vi "Day 5.vi"() -> ()   [LabVIEW 2023]
uses:
  <vilib>/Utility/error.llb/Trim Whitespace One-Sided.vi
panel:
  in  "CrateMover 9001":bool
  out "cargo":string[][](array[string])
  out "i":string
  out "giant cargo crane":string[](array[string])
  out "Top stack answer":string
  out "Moves":string[](array[string])
  in  "input":string="[B]                     [N]     [H]\n[V]         [P] [T]     [V]     [P]\n[W]     [C] [T] [S]     [H]     [N]\n[T]     [J] [Z] [M] [N] [F]     [L]\n[Q]     [W] [N] [J] [T] [Q] [R] [B]\n[N] [B] [Q] [R] [V] [F] [D] [F] [M]\n[H] [W] [S] [J] [P] [W] [L] [P] [S]\n[D] [D] [T] [F] [G] [B] [B] [H] [Z]\n 1   2   3   4   5   6   7   8   9 \n\nmove 2 from 8 to 1\nmove 4 from 9 to 8\nmove 2 from 1 to 6\nmove 7 from 4 to 2\nmove 10 from 2 to 7\nmove 2 from 1 to 6\nmove 1 from 9 to 4\nmove 1 from 4 to 1\nmove 8 from 6 to 4\nmove 7 from 1 to 8\nmove 6 from 8 to 1\nmove 1 from 4 to 1\nmove 8 from 7 to 3\nmove 2 from 5 to 2\nmove 5 from 3 to 2\nmove 5 from 2 to 1\nmove 1 from 6 to 5\nmove 2 from 2 to 6\nmove 5 from 8 to 7\nmove 12 from 7 to 4\nmove 3 from 5 to 4\nmove 2 from 6 to 4\nmove 9 from 1 to 7\nmove 4 from 3 to 7\nmove 4 from 3 to 4\nmove 3 from 1 to 7\nmove 1 from 9 to 1\nmove 1 from 1 to 4\nmove 2 from 5 to 2\nmove 1 from 3 to 7\nmove 15 from 7 to 2\nmove 4 from 7 to 9\nmove 6 from 9 to 2\nmove 2 from 8 to 3\nmove 3 from 2 to 8\nmove 1 from 7 to 6\nmove 8 from 2 to 5\nmove 2 from 8 to 4\nmove 2 from 3 to 8\nmove 9 from 5 to 9\nmove 7 from 4 to 2\nmove 1 from 8 to 6\nmove 6 from 9 to 2\nmove 3 from 9 to 7\nmove 2 from 8 to 4\nmove 7 from 2 to 6\nmove 7 from 4 to 1\nmove 3 from 1 to 8\nmove 2 from 1 to 8\nmove 4 from 8 to 2\nmove 2 from 1 to 5\nmove 19 from 2 to 7\nmove 8 from 4 to 7\nmove 18 from 7 to 1\nmove 11 from 7 to 4\nmove 15 from 1 to 7\nmove 9 from 4 to 3\nmove 2 from 3 to 1\nmove 9 from 4 to 5\nmove 1 from 8 to 1\nmove 8 from 6 to 5\nmove 3 from 2 to 5\nmove 1 from 6 to 7\nmove 4 from 4 to 3\nmove 8 from 5 to 1\nmove 13 from 1 to 6\nmove 12 from 7 to 1\nmove 12 from 6 to 3\nmove 1 from 7 to 6\nmove 1 from 7 to 5\nmove 1 from 1 to 9\nmove 1 from 3 to 1\nmove 3 from 1 to 9\nmove 12 from 3 to 8\nmove 1 from 9 to 3\nmove 1 from 6 to 8\nmove 5 from 5 to 1\nmove 1 from 6 to 2\nmove 10 from 8 to 9\nmove 13 from 9 to 2\nmove 10 from 3 to 4\nmove 1 from 8 to 9\nmove 2 from 8 to 7\nmove 1 from 3 to 1\nmove 1 from 5 to 6\nmove 13 from 2 to 5\nmove 1 from 9 to 2\nmove 7 from 1 to 4\nmove 2 from 2 to 5\nmove 2 from 7 to 8\nmove 1 from 6 to 8\nmove 10 from 5 to 8\nmove 3 from 7 to 2\nmove 4 from 1 to 4\nmove 12 from 4 to 2\nmove 10 from 5 to 3\nmove 6 from 2 to 1\nmove 2 from 4 to 8\nmove 3 from 4 to 8\nmove 6 from 1 to 7\nmove 1 from 7 to 5\nmove 12 from 8 to 2\nmove 3 from 4 to 9\nmove 1 from 4 to 3\nmove 2 from 9 to 6\nmove 2 from 6 to 8\nmove 1 from 1 to 3\nmove 8 from 2 to 6\nmove 4 from 1 to 8\nmove 12 from 2 to 3\nmove 4 from 6 to 8\nmove 10 from 8 to 3\nmove 14 from 3 to 8\nmove 5 from 5 to 8\nmove 1 from 7 to 8\nmove 5 from 3 to 5\nmove 4 from 7 to 2\nmove 2 from 6 to 1\nmove 4 from 3 to 7\nmove 4 from 5 to 1\nmove 21 from 8 to 6\nmove 7 from 3 to 2\nmove 1 from 5 to 1\nmove 4 from 8 to 9\nmove 16 from 6 to 1\nmove 1 from 8 to 4\nmove 5 from 9 to 2\nmove 7 from 1 to 7\nmove 10 from 1 to 3\nmove 1 from 4 to 2\nmove 6 from 6 to 5\nmove 6 from 1 to 4\nmove 4 from 7 to 9\nmove 1 from 6 to 5\nmove 5 from 7 to 6\nmove 3 from 6 to 8\nmove 1 from 7 to 6\nmove 6 from 4 to 8\nmove 4 from 8 to 3\nmove 4 from 8 to 4\nmove 17 from 2 to 1\nmove 8 from 3 to 4\nmove 5 from 4 to 3\nmove 10 from 1 to 5\nmove 11 from 3 to 5\nmove 1 from 7 to 9\nmove 3 from 6 to 4\nmove 9 from 4 to 9\nmove 7 from 1 to 3\nmove 1 from 4 to 8\nmove 7 from 5 to 4\nmove 18 from 5 to 1\nmove 13 from 1 to 6\nmove 1 from 1 to 5\nmove 1 from 1 to 6\nmove 2 from 3 to 1\nmove 1 from 3 to 1\nmove 5 from 1 to 6\nmove 4 from 5 to 8\nmove 2 from 4 to 9\nmove 1 from 1 to 9\nmove 6 from 3 to 8\nmove 1 from 4 to 5\nmove 10 from 8 to 7\nmove 16 from 6 to 7\nmove 1 from 5 to 4\nmove 1 from 7 to 2\nmove 2 from 2 to 6\nmove 2 from 8 to 5\nmove 5 from 4 to 9\nmove 2 from 5 to 9\nmove 7 from 9 to 8\nmove 2 from 6 to 9\nmove 4 from 8 to 9\nmove 7 from 9 to 7\nmove 13 from 9 to 5\nmove 10 from 5 to 1\nmove 3 from 8 to 4\nmove 5 from 1 to 3\nmove 3 from 5 to 6\nmove 3 from 9 to 7\nmove 1 from 1 to 7\nmove 2 from 1 to 3\nmove 1 from 6 to 1\nmove 4 from 3 to 8\nmove 1 from 8 to 9\nmove 1 from 8 to 7\nmove 1 from 8 to 4\nmove 1 from 9 to 7\nmove 1 from 8 to 5\nmove 2 from 4 to 3\nmove 4 from 6 to 3\nmove 1 from 5 to 1\nmove 1 from 6 to 4\nmove 2 from 4 to 5\nmove 1 from 4 to 6\nmove 1 from 6 to 4\nmove 30 from 7 to 3\nmove 1 from 5 to 1\nmove 6 from 7 to 3\nmove 2 from 1 to 7\nmove 2 from 1 to 2\nmove 2 from 2 to 1\nmove 1 from 4 to 9\nmove 3 from 1 to 2\nmove 1 from 9 to 5\nmove 2 from 7 to 1\nmove 1 from 7 to 3\nmove 1 from 1 to 9\nmove 1 from 5 to 8\nmove 1 from 1 to 2\nmove 1 from 7 to 3\nmove 1 from 9 to 4\nmove 18 from 3 to 4\nmove 1 from 5 to 9\nmove 1 from 9 to 6\nmove 1 from 2 to 7\nmove 1 from 8 to 7\nmove 1 from 6 to 3\nmove 1 from 7 to 2\nmove 14 from 4 to 6\nmove 1 from 7 to 6\nmove 15 from 6 to 4\nmove 20 from 3 to 1\nmove 5 from 4 to 9\nmove 5 from 4 to 2\nmove 15 from 1 to 7\nmove 11 from 7 to 9\nmove 2 from 7 to 6\nmove 1 from 6 to 4\nmove 1 from 6 to 3\nmove 2 from 7 to 8\nmove 10 from 4 to 3\nmove 15 from 9 to 3\nmove 1 from 9 to 7\nmove 29 from 3 to 6\nmove 3 from 1 to 6\nmove 1 from 8 to 4\nmove 2 from 4 to 3\nmove 1 from 8 to 9\nmove 4 from 6 to 1\nmove 20 from 6 to 2\nmove 5 from 1 to 9\nmove 3 from 6 to 2\nmove 4 from 6 to 3\nmove 4 from 3 to 1\nmove 4 from 1 to 4\nmove 3 from 4 to 8\nmove 6 from 3 to 4\nmove 6 from 2 to 6\nmove 1 from 7 to 1\nmove 3 from 6 to 8\nmove 6 from 9 to 3\nmove 1 from 1 to 4\nmove 1 from 1 to 7\nmove 3 from 4 to 5\nmove 2 from 6 to 4\nmove 2 from 5 to 6\nmove 4 from 8 to 7\nmove 1 from 5 to 6\nmove 1 from 8 to 4\nmove 1 from 8 to 4\nmove 2 from 4 to 9\nmove 4 from 7 to 8\nmove 4 from 4 to 3\nmove 1 from 7 to 9\nmove 4 from 8 to 6\nmove 1 from 3 to 4\nmove 1 from 3 to 5\nmove 2 from 4 to 7\nmove 4 from 6 to 3\nmove 2 from 9 to 1\nmove 2 from 7 to 4\nmove 1 from 5 to 1\nmove 1 from 3 to 4\nmove 1 from 9 to 3\nmove 4 from 4 to 5\nmove 2 from 5 to 3\nmove 1 from 5 to 7\nmove 1 from 5 to 8\nmove 2 from 6 to 4\nmove 3 from 1 to 3\nmove 21 from 3 to 5\nmove 3 from 6 to 1\nmove 1 from 7 to 1\nmove 4 from 2 to 6\nmove 1 from 8 to 2\nmove 10 from 2 to 4\nmove 4 from 1 to 2\nmove 1 from 6 to 5\nmove 2 from 6 to 9\nmove 7 from 4 to 9\nmove 1 from 6 to 5\nmove 3 from 9 to 4\nmove 6 from 2 to 8\nmove 3 from 9 to 1\nmove 8 from 4 to 3\nmove 1 from 9 to 4\nmove 21 from 5 to 7\nmove 1 from 1 to 3\nmove 2 from 9 to 6\nmove 14 from 7 to 1\nmove 2 from 4 to 1\nmove 2 from 8 to 7\nmove 1 from 8 to 2\nmove 11 from 2 to 9\nmove 8 from 9 to 6\nmove 4 from 7 to 1\nmove 1 from 7 to 4\nmove 2 from 3 to 5\nmove 1 from 1 to 6\nmove 1 from 8 to 2\nmove 3 from 7 to 5\nmove 6 from 1 to 7\nmove 1 from 8 to 7\nmove 1 from 4 to 5\nmove 4 from 6 to 5\nmove 6 from 7 to 6\nmove 3 from 9 to 1\nmove 1 from 7 to 3\nmove 11 from 5 to 1\nmove 1 from 5 to 2\nmove 9 from 6 to 4\nmove 1 from 7 to 3\nmove 2 from 6 to 1\nmove 1 from 2 to 1\nmove 1 from 2 to 6\nmove 14 from 1 to 5\nmove 1 from 8 to 4\nmove 10 from 1 to 5\nmove 3 from 5 to 1\nmove 8 from 3 to 8\nmove 16 from 5 to 7\nmove 2 from 1 to 9\nmove 3 from 8 to 1\nmove 1 from 2 to 4\nmove 6 from 7 to 4\nmove 3 from 5 to 8\nmove 2 from 3 to 6\nmove 7 from 1 to 7\nmove 14 from 4 to 3\nmove 9 from 7 to 8\nmove 2 from 4 to 1\nmove 9 from 8 to 4\nmove 7 from 8 to 2\nmove 6 from 1 to 8\nmove 1 from 9 to 7\nmove 1 from 1 to 6\nmove 1 from 9 to 6\nmove 1 from 5 to 9\nmove 1 from 5 to 3\nmove 9 from 4 to 9\nmove 3 from 3 to 6\nmove 8 from 6 to 3\nmove 1 from 2 to 9\nmove 8 from 9 to 8\nmove 6 from 2 to 9\nmove 2 from 6 to 1\nmove 7 from 8 to 6\nmove 2 from 9 to 6\nmove 8 from 7 to 8\nmove 1 from 4 to 5\nmove 9 from 3 to 5\nmove 2 from 1 to 4\nmove 1 from 7 to 4\nmove 2 from 4 to 3\nmove 11 from 8 to 1\nmove 1 from 4 to 7\nmove 1 from 7 to 8\nmove 5 from 1 to 3\nmove 4 from 6 to 4\nmove 2 from 4 to 8\nmove 1 from 4 to 8\nmove 7 from 8 to 9\nmove 1 from 8 to 9\nmove 1 from 8 to 5\nmove 18 from 3 to 2\nmove 17 from 2 to 7\nmove 6 from 5 to 4\nmove 1 from 2 to 5\nmove 4 from 4 to 6\nmove 4 from 6 to 9\nmove 15 from 7 to 9\nmove 2 from 1 to 6\nmove 2 from 7 to 9\nmove 28 from 9 to 2\nmove 1 from 6 to 7\nmove 4 from 6 to 9\nmove 3 from 1 to 7\nmove 2 from 6 to 3\nmove 1 from 4 to 7\nmove 8 from 9 to 5\nmove 13 from 5 to 3\nmove 1 from 5 to 7\nmove 3 from 9 to 4\nmove 8 from 3 to 7\nmove 28 from 2 to 5\nmove 1 from 9 to 8\nmove 4 from 3 to 4\nmove 4 from 7 to 5\nmove 2 from 3 to 9\nmove 21 from 5 to 4\nmove 1 from 5 to 7\nmove 1 from 3 to 5\nmove 3 from 5 to 7\nmove 1 from 1 to 3\nmove 3 from 7 to 3\nmove 5 from 7 to 6\nmove 10 from 4 to 8\nmove 6 from 5 to 4\nmove 1 from 9 to 3\nmove 15 from 4 to 5\nmove 10 from 4 to 7\nmove 3 from 3 to 7\nmove 1 from 3 to 4\nmove 1 from 3 to 4\nmove 7 from 5 to 1\nmove 2 from 4 to 7\nmove 1 from 9 to 2\nmove 2 from 6 to 9\nmove 1 from 5 to 3\nmove 1 from 3 to 8\nmove 10 from 7 to 9\nmove 2 from 8 to 1\nmove 9 from 9 to 2\nmove 1 from 4 to 3\nmove 9 from 8 to 7\nmove 1 from 2 to 8\nmove 5 from 5 to 4\nmove 1 from 3 to 2\nmove 5 from 4 to 3\nmove 3 from 5 to 9\nmove 6 from 7 to 3\nmove 1 from 6 to 5\nmove 5 from 9 to 7\nmove 2 from 5 to 6\nmove 3 from 6 to 7\nmove 4 from 1 to 4\nmove 6 from 2 to 7\nmove 17 from 7 to 5\nmove 1 from 6 to 1\nmove 5 from 3 to 6\nmove 10 from 7 to 2\nmove 1 from 8 to 4\nmove 1 from 9 to 8\nmove 3 from 4 to 1\nmove 1 from 7 to 4\nmove 5 from 5 to 9\nmove 2 from 8 to 7\nmove 3 from 3 to 7\nmove 4 from 2 to 3\nmove 3 from 4 to 6\nmove 7 from 5 to 8\nmove 7 from 2 to 8\nmove 4 from 9 to 8\nmove 12 from 8 to 3\nmove 17 from 3 to 2\nmove 1 from 7 to 9\nmove 1 from 3 to 9\nmove 3 from 9 to 1\nmove 2 from 5 to 1\nmove 1 from 3 to 5\nmove 4 from 5 to 8\nmove 6 from 8 to 1\nmove 17 from 2 to 3\nmove 13 from 3 to 2\nmove 1 from 3 to 9\nmove 1 from 8 to 4\nmove 1 from 4 to 8\nmove 1 from 9 to 1\nmove 2 from 7 to 2\nmove 8 from 6 to 2\nmove 2 from 7 to 5\nmove 9 from 1 to 3\nmove 13 from 2 to 9\nmove 6 from 1 to 4\nmove 6 from 4 to 5\nmove 3 from 8 to 1\nmove 2 from 1 to 8\nmove 8 from 5 to 7\nmove 2 from 3 to 1\nmove 9 from 3 to 1\nmove 3 from 8 to 2\nmove 1 from 1 to 9\nmove 1 from 3 to 9\nmove 6 from 7 to 3\nmove 4 from 2 to 7\nmove 14 from 1 to 6\nmove 2 from 3 to 9\nmove 3 from 3 to 7\nmove 6 from 2 to 1\nmove 2 from 1 to 2\nmove 9 from 6 to 3\nmove 11 from 9 to 5\nmove 9 from 7 to 6\nmove 6 from 6 to 2\nmove 1 from 1 to 8\nmove 5 from 9 to 4\nmove 1 from 8 to 5\nmove 9 from 2 to 7\nmove 10 from 5 to 8\n"
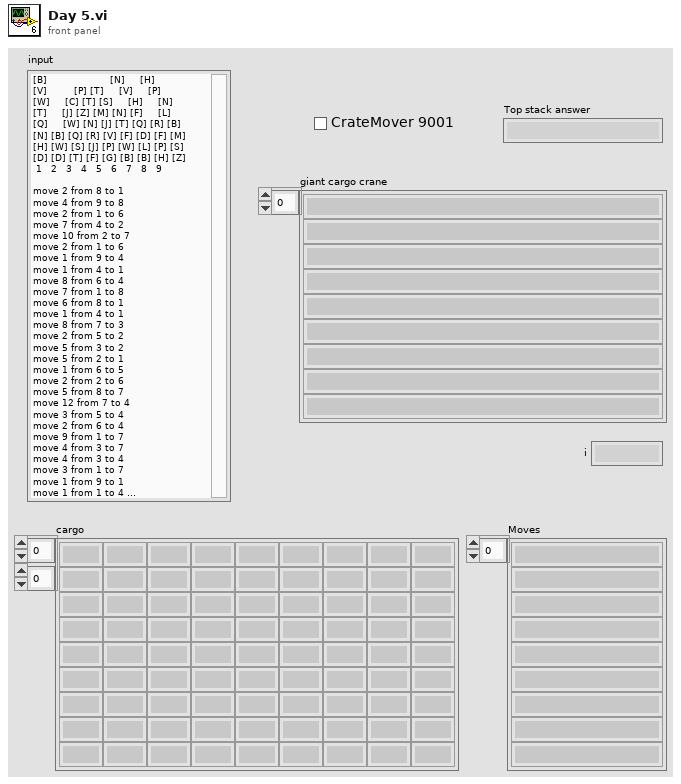
[diagram p1: front panel]
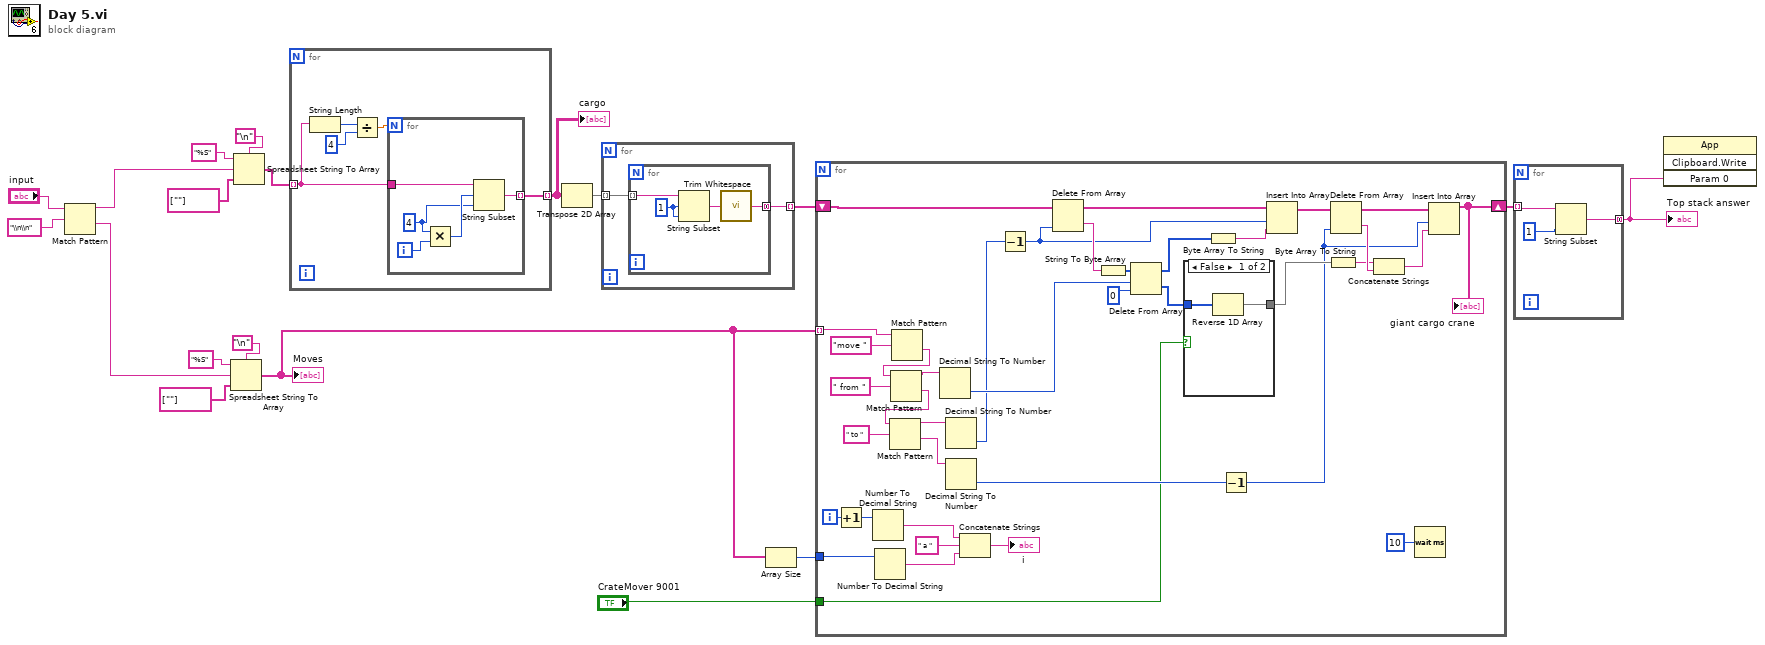
[diagram p0: block diagram]
diagram:
  n1 = Match Pattern(string="input", regular expression="\\n\\n") -> (before substring=w11:string, after substring=w10:string)  [unwired: 1 in, 2 out]
  n2 = Spreadsheet String To Array(delimiter (Tab)="\n", format string="%S", spreadsheet string=w10, array type (2D Dbl)=string[] [""]) -> (array=w5:string[])
  "Moves" <- w5
  n3 = Spreadsheet String To Array(delimiter (Tab)="\n", format string="%S", spreadsheet string=w11, array type (2D Dbl)=string[] [""]) -> (array=w9:string[])
  n4 = for {
    tunnel: w9 -> [w21] mode=indexing
    tunnel: [w20] -> w2 mode=indexing
    n5 = String Length(string=w21) -> (length=w24:i32)
    n6 = Divide(x=w24, y=4) -> (x/y=w22:dbl)
    n7 = for {
      N: w22 -> [_]
      tunnel: w21 -> [w26]
      tunnel: [w25] -> w20 mode=indexing
      i -> [w29]
      w27 = 4 ("x")
      n8 = Multiply(x=w27, y=w29) -> (x*y=w28:i32)
      n9 = String Subset(string=w26, offset (0)=w28, length (rest)=w27) -> (substring=w25:string)
    }
  }
  "cargo" <- w2
  n10 = Transpose 2D Array(2D array=w2) -> (transposed array=w8:string[][])
  n11 = for {
    tunnel: w8 -> [w31] mode=indexing
    tunnel: [w30] -> w3 mode=indexing
    n12 = for {
      tunnel: w31 -> [w35] mode=indexing
      tunnel: [w33] -> w30 mode=concatenating
      w32 = 1 ("offset (0)")
      n13 = String Subset(string=w35, offset (0)=w32, length (rest)=w32) -> (substring=w34:string)
      n14 = call <vilib>:"Trim Whitespace.vi"("string"=w34) -> ("trimmed string"=w33:string)  [unwired: 1 in]
    }
  }
  n15 = Array Size(array=w5) -> (size(s)=w4:i32)
  n16 = for {
    tunnel: w5 -> [w64] mode=indexing
    shift-right: [w46] -> w7
    shift-left: w3 -> [w47]
    tunnel: w4 -> [w42]
    tunnel: "CrateMover 9001" -> [w36]
    i -> [w44]
    n17 = Increment(x=w44) -> (x+1=w38:i32)
    n18 = Number To Decimal String(number=w38) -> (decimal integer string=w43:string)  [unwired: 1 in]
    n19 = Number To Decimal String(number=w42) -> (decimal integer string=w41:string)  [unwired: 1 in]
    n20 = Match Pattern(string=w64, regular expression="move ") -> (after substring=w69:string)  [unwired: 1 in, 3 out]
    n21 = Match Pattern(string=w69, regular expression=" from ") -> (before substring=w70:string, after substring=w67:string)  [unwired: 1 in, 2 out]
    n22 = Match Pattern(string=w67, regular expression=" to ") -> (before substring=w71:string, after substring=w72:string)  [unwired: 1 in, 2 out]
    n23 = Decimal String To Number(string=w70) -> (number=w60:i32)  [unwired: 2 in, 1 out]
    n24 = Decimal String To Number(string=w71) -> (number=w56:i32)  [unwired: 2 in, 1 out]
    n25 = Decimal String To Number(string=w72) -> (number=w73:i32)  [unwired: 2 in, 1 out]
    n26 = Concatenate Strings(w43, " a " ("string"), w41) -> (→"i":string)
    n27 = Decrement(x=w56) -> (x-1=w55:i32)
    n28 = Delete From Array(array=w47, index=w55) -> (deleted portion=w62:string, array with subset deleted=w63:string[])  [unwired: 1 in]
    n29 = String To Byte Array(string=w62) -> (unsigned byte array=w61:u8[])
    n30 = Delete From Array(array=w61, length=w60, index=0) -> (deleted portion=w37:u8[], array with subset deleted=w59:u8[])
    n31 = case shown="False" w36 {
      tunnel: [w75 w76] -> w58
      tunnel: w37 -> [w74 w76]
      frame False {
        n32 = Reverse 1D Array(array=w74) -> (reversed array=w75:u8[])
      }
      frame True {
      }
    }
    n33 = Byte Array To String(unsigned byte array=w59) -> (string=w57:string)
    n34 = Decrement(x=w73) -> (x-1=w48:i32)
    n35 = Insert Into Array(array=w63, index=w55, new element=w57) -> (w53:string[])
    n36 = Byte Array To String(unsigned byte array=w58) -> (string=w51:string)
    n37 = Delete From Array(array=w53, index=w48) -> (deleted portion=w52:string, array with subset deleted=w50:string[])  [unwired: 1 in]
    n38 = Concatenate Strings(w51, w52) -> (w49:string)
    n39 = Wait (ms)(milliseconds to wait=u32 10) -> ()  [unwired: 1 out]
    n40 = Insert Into Array(array=w50, index=w48, new element=w49) -> (w46:string[])
    "giant cargo crane" <- w46
  }
  n41 = for {
    tunnel: w7 -> [w79] mode=indexing
    tunnel: [w77] -> w6 mode=concatenating
    n42 = String Subset(string=w79, length (rest)=1 ("length (rest)")) -> (substring=w77:string)  [unwired: 1 in]
  }
  "Top stack answer" <- w6
  n43 = invoke class="App" method="Clipboard.Write"("Param 0"=w6) -> ()  [unwired: 3 in, 4 out]
